vi "FindNullSpace (SubVI).vi"(0 "Matrix":T1) -> (1 "Null":T1, 2 "rank":i32)   [LabVIEW 2021]
uses:
  <vilib>/Analysis/Matrix/Datatypes/RealMatrix.ctl
  <vilib>/Analysis/7linalg.llb/SVD Option.ctl
  <vilib>/Analysis/_algsub.llb/Real Matrix Rank.vi
  <vilib>/Analysis/7linalg.llb/Real SVD Decomposition.vi
  <vilib>/Analysis/NI_AALPro.lvlib
  <vilib>/Analysis/Matrix/NI_Matrix.lvlib
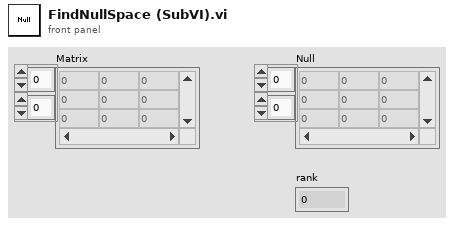
[diagram p1: front panel]
types:
  T1 = typedef "NI_Matrix.lvlib/RealMatrix.ctl" = dbl[][]
  T2 = typedef "NI_AALPro.lvlib/SVD Option.ctl" = u16
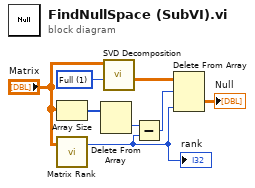
[diagram p0: block diagram]
diagram:
  w6 = T2 1 items=["Thin", "Full"] ("SVD option")
  n1 = Array Size(array="Matrix") -> (size(s)=w2:i32[])
  n2 = call-poly <vilib>:"Matrix Rank.vi"("Input Matrix"="Matrix") -> ("rank"=w4:i32)  [unwired: 1 in, 1 out]
  "rank" <- w4
  n3 = Delete From Array(array=w2) -> (deleted portion=w3:i32)  [unwired: 2 in, 1 out]
  n4 = call-poly <vilib>:"SVD Decomposition.vi"("SVD option"=w6, "A"="Matrix") -> ("Matrix V"=w1:T1)  [unwired: 5 in, 4 out]
  n5 = Subtract(x=w3, y=w4) -> (x-y=w5:i32)
  n6 = Delete From Array(array=w1, length=w5, index (col)=w4) -> (deleted portion=→"Null":T1)  [unwired: 1 in, 1 out]
